vi "set_no_proxy.vi"(8 "error in (no error)":errorcluster, 11 "ClientBuilder in":refnum<class "ClientBuilder.lvclass">) -> (0 "error out":errorcluster, 2 "success":bool, 3 "ClientBuilder out":refnum<class "ClientBuilder.lvclass">)   [LabVIEW 2020, in "reqwest.lvlib" / "ClientBuilder.lvclass"]
uses:
  ClientBuilder.lvclass
  ClientBuilder.lvclass/ClientBuilder.ctl
  lv_reqwest_64.dll
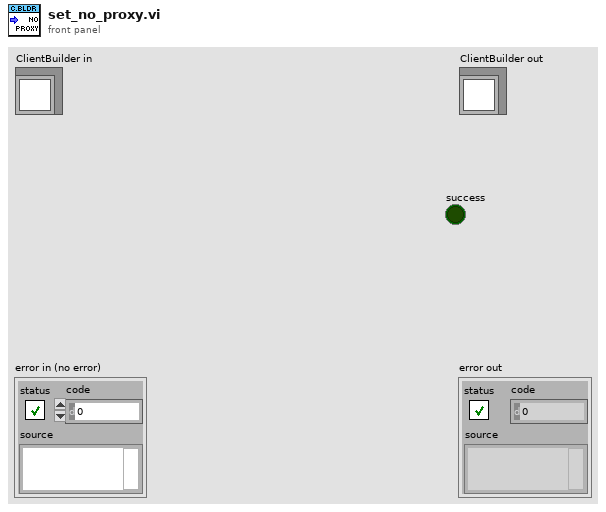
[diagram p1: front panel]
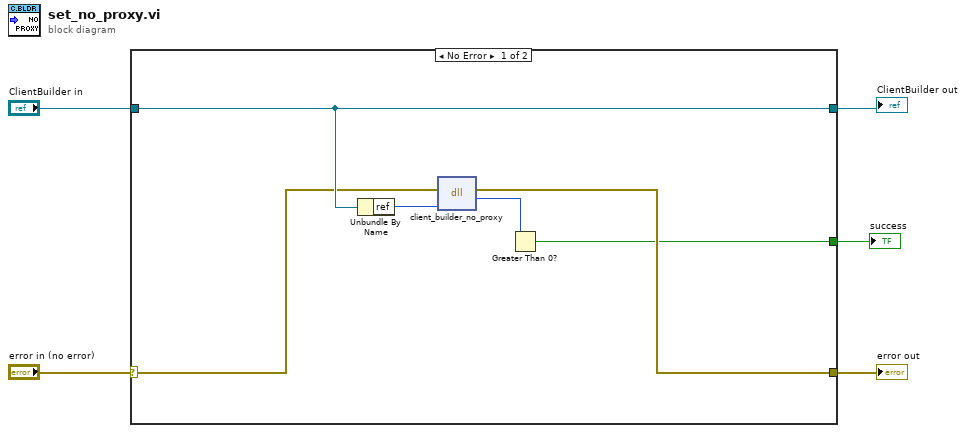
[diagram p0: block diagram]
diagram:
  n1 = case shown="No Error" "error in (no error)" {
    selector: "error in (no error)" -> [w8 w12]
    tunnel: "ClientBuilder in" -> [w9 w13]
    tunnel: [w11 w12] -> w2
    tunnel: [w9 w13] -> w3
    tunnel: [w6 _] -> w1
    frame No Error {
      n2 = Unbundle By Name(w9) -> ("ref"=w10:u64)
      n3 = dll-call lib="C:/Projects/vipm-desktop/source/submodules/reqwest-rs-labview/lv_src/lv_reqwest_*.*" fn="client_builder_no_proxy"(error in=w8, "client_builder_ref"=w10) -> (error out=w11:errorcluster, "success"=w7:u8)  [unwired: 3 in, 1 out]
      n4 = Greater Than 0?(x=w7) -> (x > 0?=w6:bool)
    }
    frame Error {
    }
  }
  "error out" <- w2
  "ClientBuilder out" <- w3
  "success" <- w1
